vi "Start.vi"(8 "error in (no error)":errorcluster, 11 "Thermometer DAQmx in":refnum<class "Thermometer DAQmx.lvclass">) -> (0 "error out":errorcluster, 3 "Thermometer DAQmx out":refnum<class "Thermometer DAQmx.lvclass">)   [LabVIEW 2023, in "Thermometer.lvlib" / "Thermometer DAQmx.lvlib" / "Thermometer DAQmx.lvclass"]
uses:
  Thermometer DAQmx.lvclass
  Thermometer DAQmx.lvclass/Thermometer DAQmx.ctl
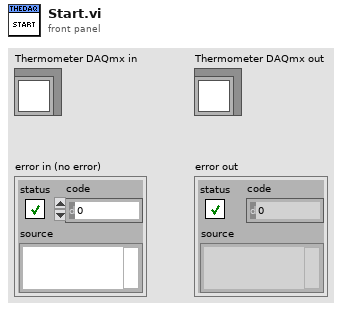
[diagram p1: front panel]
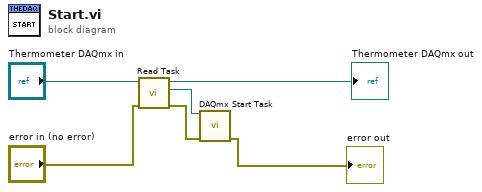
[diagram p0: block diagram]
diagram:
  n1 = call-dynamic "Read Task.vi"("error in (no error)"="error in (no error)", "Thermometer DAQmx in"="Thermometer DAQmx in") -> ("error out"=w3:errorcluster, "Task"=w4:refnum<k21>, "Thermometer DAQmx out"=→"Thermometer DAQmx out":refnum<class "Thermometer DAQmx.lvclass">)  [unwired: 7 in]
  n2 = call <vilib>:"DAQmx Start Task.vi"("task/channels in"=w4, "error in"=w3) -> ("error out"=→"error out":errorcluster)  [unwired: 12 in, 1 out]
